vi "Connect.vi"(7 "Address":string, 8 "error in":errorcluster, 9 "RawSocket Handler in":refnum<class "RawSocket Handler.lvclass">) -> (2 "error out":errorcluster, 3 "RawSocket Handler out":refnum<class "RawSocket Handler.lvclass">)   [LabVIEW 2020, in "wamplv.lvlib" / "RawSocket Handler.lvclass"]
uses:
  RawSocket Handler.lvclass
  C:/local/wamplv/CommHandlerBase/CommHandlerBase.lvclass
  <vilib>/LabVIEW Open Source Project/OpenURI/uri/URI.lvclass/URI.ctl
  RawSocket Handler.lvclass/RawSocket Handler.ctl
  <vilib>/LabVIEW Open Source Project/OpenURI/uri/URI.lvclass
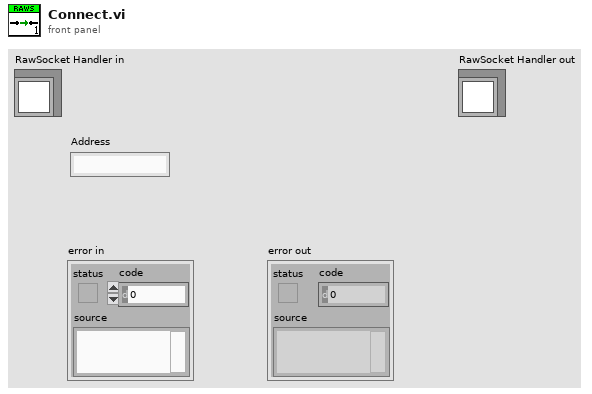
[diagram p1: front panel]
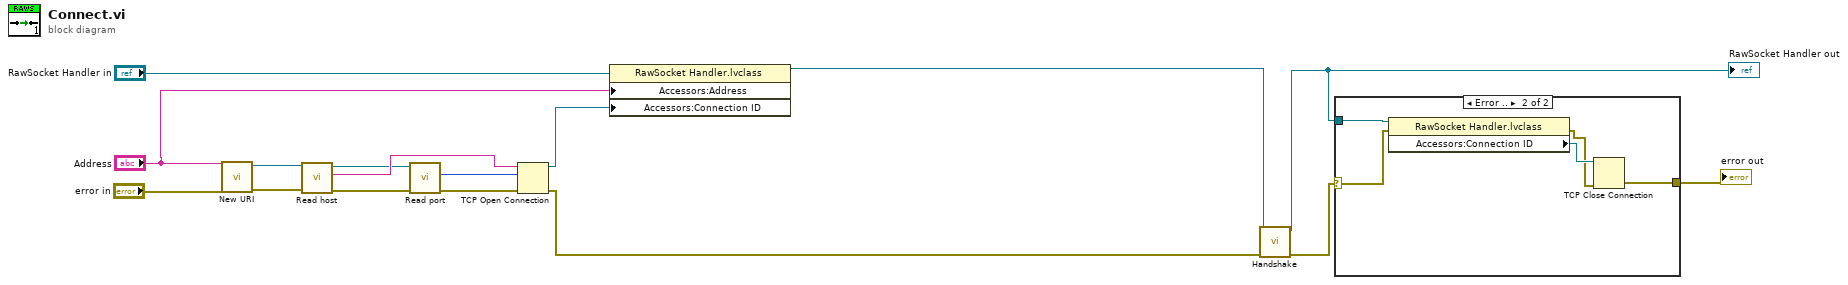
[diagram p0: block diagram]
diagram:
  n1 = call <vilib>:"New URI.vi"("error in (no error)"="error in", "URI"="Address") -> ("error out"=w13:errorcluster, "URI"=w14:refnum<class "URI.lvclass">)  [unwired: 8 in]
  n2 = call <vilib>:"Read host.vi"("error in (no error)"=w13, "URI in"=w14) -> ("error out"=w11:errorcluster, "host"=w12:string, "URI out"=w10:refnum<class "URI.lvclass">)  [unwired: 7 in]
  n3 = call <vilib>:"Read port.vi"("error in (no error)"=w11, "URI in"=w10) -> ("error out"=w6:errorcluster, "port"=w9:u16)  [unwired: 7 in, 1 out]
  n4 = TCP Open Connection(address=w12, remote port or service name=w9, error in (no error)=w6) -> (connection ID=w4:refnum<k5>, error out=w2:errorcluster)  [unwired: 2 in]
  n5 = property class="RawSocket Handler.lvclass"(reference="RawSocket Handler in", "Accessors:Address"="Address", "Accessors:Connection ID"=w4) -> (reference out=w7:refnum<class "RawSocket Handler.lvclass">)  [unwired: 1 in, 1 out]
  n6 = call "Handshake.vi"("error in"=w2, "RawSocket Handler in"=w7) -> ("error out"=w5:errorcluster, "RawSocket Handler out"=w1:refnum<class "RawSocket Handler.lvclass">)  [unwired: 8 in]
  "RawSocket Handler out" <- w1
  n7 = case shown="Error .." w5 {
    selector: w5 -> [w17 w19]
    tunnel: [w17 w22] -> w3
    tunnel: w1 -> [_ w21]
    frame No Error {
    }
    frame Error {
      n8 = property class="RawSocket Handler.lvclass"(reference=w21, error in=w19) -> (error out=w18:errorcluster, "Accessors:Connection ID"=w20:refnum<k5>)  [unwired: 1 out]
      n9 = TCP Close Connection(connection ID=w20, error in (no error)=w18) -> (error out=w22:errorcluster)  [unwired: 1 in, 1 out]
    }
  }
  "error out" <- w3
